vi "Makepath2017.vi"(0 "text to save":string, 1 "File name, format \\filename":string) -> ()   [LabVIEW 2017]
panel:
  out "date string":string
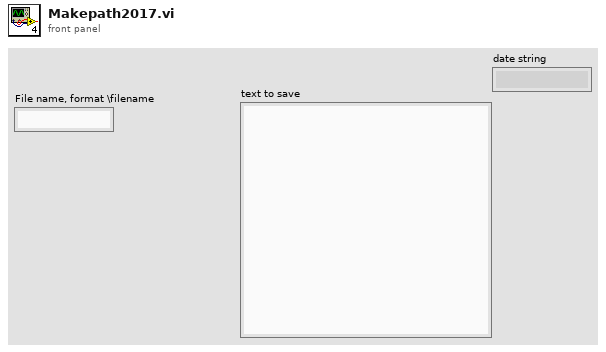
[diagram p1: front panel]
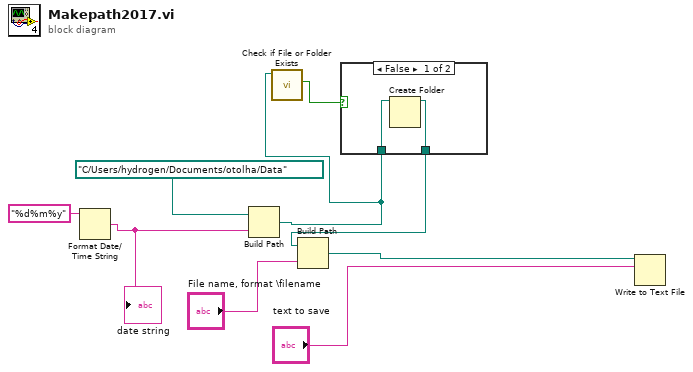
[diagram p0: block diagram]
diagram:
  n1 = Format Date/Time String(time format string (%c)="%d%m%y") -> (date/time string=w6:string)  [unwired: 2 in]
  "date string" <- w6
  n2 = Build Path(base path=path "C:/Users/hydrogen/Documents/otolha/Data", name or relative path=w6) -> (appended path=w1:path)
  n3 = call <vilib>:"Check if File or Folder Exists.vi"("path"=w1) -> ("file or folder exists?"=w2:bool)  [unwired: 8 in, 2 out]
  n4 = case shown="False" w2 {
    tunnel: w1 -> [w11 w12]
    tunnel: [w10 w12] -> w3
    frame False {
      n5 = Create Folder(path (use dialog)=w11) -> (created path=w10:path)  [unwired: 2 in, 2 out]
    }
    frame True {
    }
  }
  n6 = Build Path(base path=w3, name or relative path="File name, format \\filename") -> (appended path=w4:path)
  n7 = Write to Text File(file (use dialog)=w4, text="text to save") -> ()  [unwired: 2 in, 3 out]
